vi "Advanced Functionality with Attributes.vi"() -> ()   [LabVIEW 2023]
doc: "The Advanced Functionality with Attributes example allows the user to view a camera's current attributes and settings, update attribute settings, acquire images continuously, and display the images in an image control. Note that the writeability of some attributes changes while acquiring and this is denoted by disabling the attribute."
uses:
  <vilib>/userdefined/High Color/IMAQdx.ctl
  <vilib>/vision/driver/IMAQdx.llb/IMAQdx Buffer Number Mode.ctl
  <vilib>/vision/driver/NI_Vision_Acquisition_Software.lvlib
panel:
  out "Frame Rate":dbl format="%#.2g"
  in  "Tab Control":T1(tab)
  in  "U32 Value Control":u32(slide) min=1 max=32768 step=1 scale=1.0..32768.0
  in  "DBL Value Control":dbl(slide) min=-100.0 max=100.0 step=1.0 scale=-100.0..100.0
  in  "String Value Control":string
  in  "Enum Value Control":u32(ring) items=["Mono8", "Mono10", "Mono12", "Mono14", "Mono16", "YUV422Packed"]
  in  "Boolean Value Control":bool
  in  "Command Value Control":bool
  in  "Grab":bool
  out "Tooltip":string
  out "Units":string
  in  "Attribute Tree":string(tree)
  out "Image":T2(plugin-control)
  out "Buffer Number":u32
  in  "Camera Name":refnum<k21> caption="IMAQdx Session"
  in  "Stop":bool
  # "Overview: Demonstrates how to view a camera's current attributes and settings, update attribute settings, acquire images continuously, and display the images in an image control.\nRequirements: Vision Acquisition Software\nInstructions: \n1. Select the Camera Name\n2. Run the VI\n3. Select various attributes in the tree to view the settings for the attribute.\n4. Press the Start Grab button and notice some attributes are no longer writeable; they are disabled. This is a property of attributes that can change as the acquisition state changes or other attribute values change."
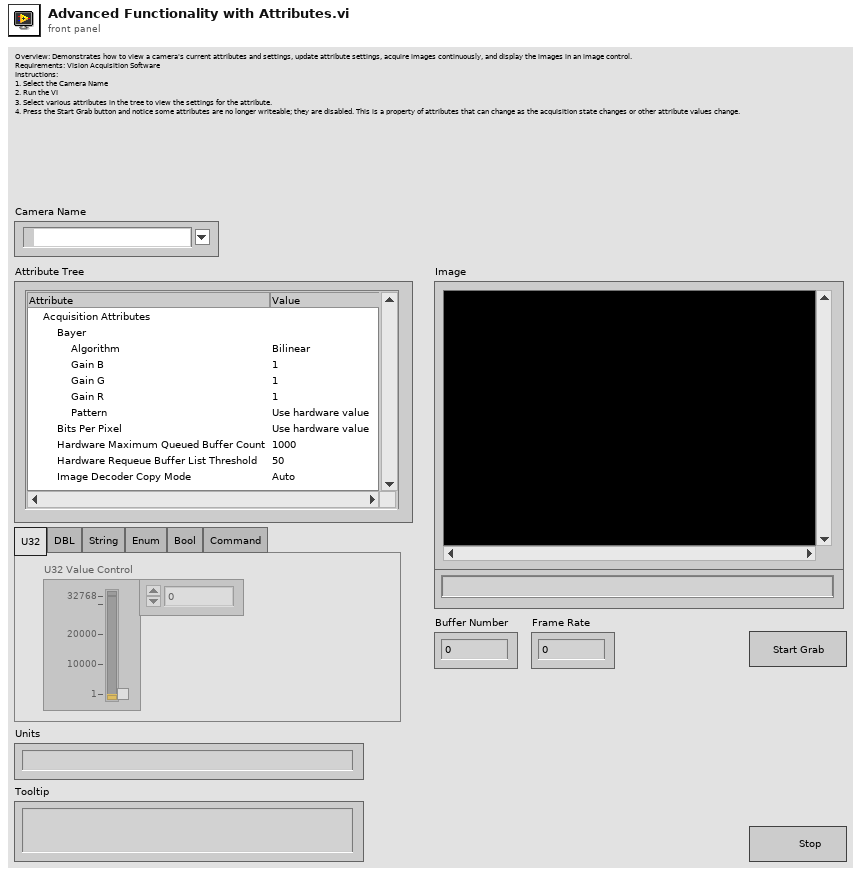
[diagram p1: front panel]
types:
  T1 = enum32{"U32", "DBL", "String", "Enum", "Bool", "Command"}
  T2 = typedef "IMAQ Image.ctl" = refnum<image>
  T3 = typedef "IMAQdx.ctl" = refnum<k21>
  T4 = cluster{"Tab Control":refnum<vi>, "U32 Value Control":refnum<vi>, "DBL Value Control":refnum<vi>, "String Value Control":refnum<vi>, "Enum Value Control":refnum<vi>, "Boolean Value Control":refnum<vi>, "Command Value Control":refnum<vi>}
  T5 = typedef "NI_Vision_Acquisition_Software.lvlib/IMAQdx Buffer Number Mode.ctl" = enum32{"Next", "Last", "Buffer Number", "Every", "Last New"}
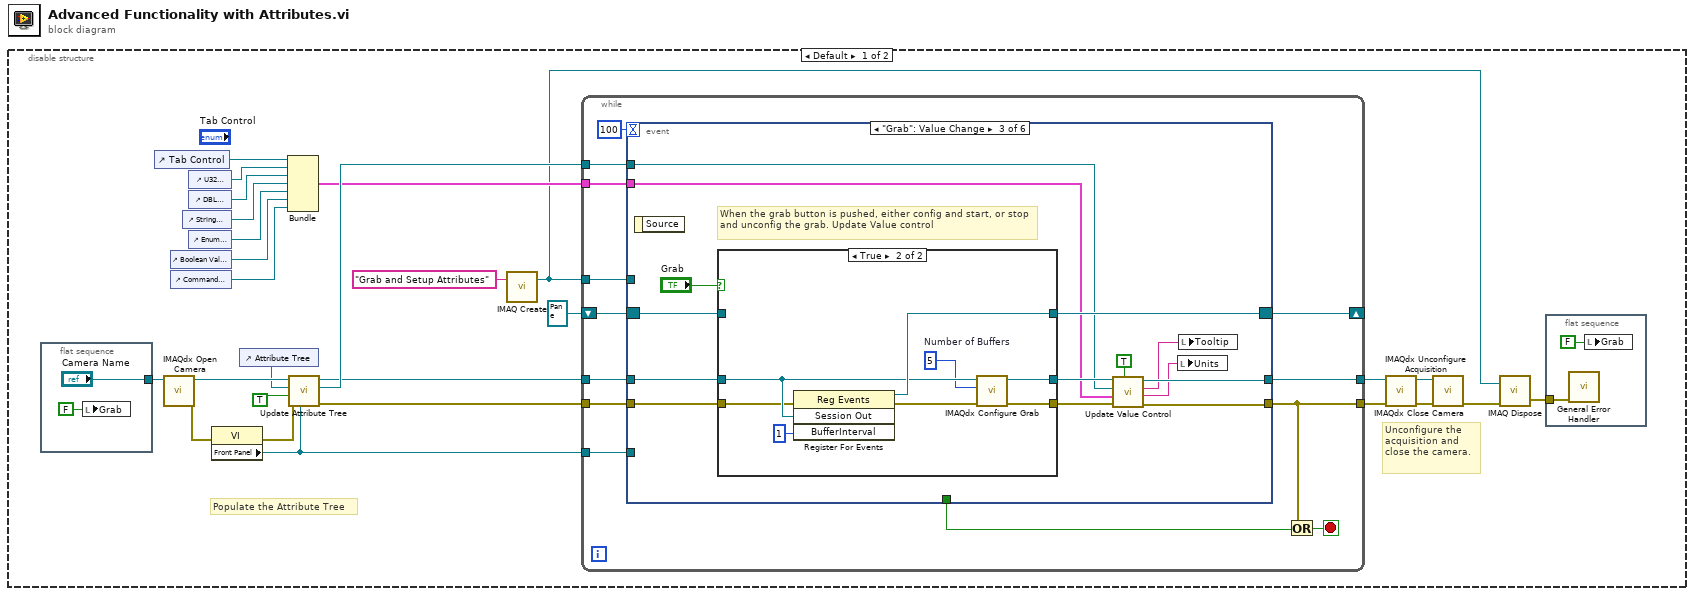
[diagram p0: block diagram]
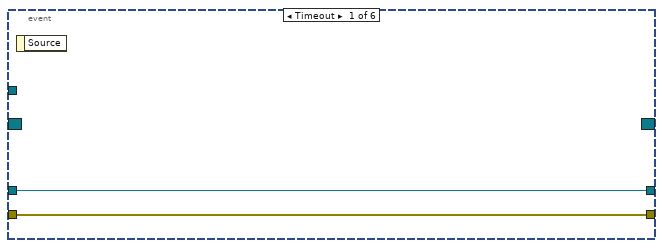
[diagram p2: hidden frame]
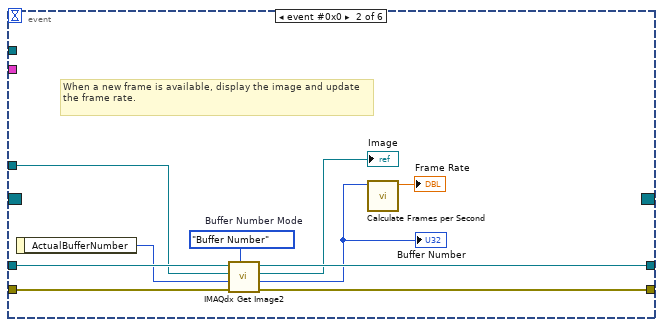
[diagram p3: hidden frame]
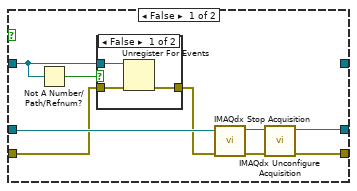
[diagram p4: hidden frame]
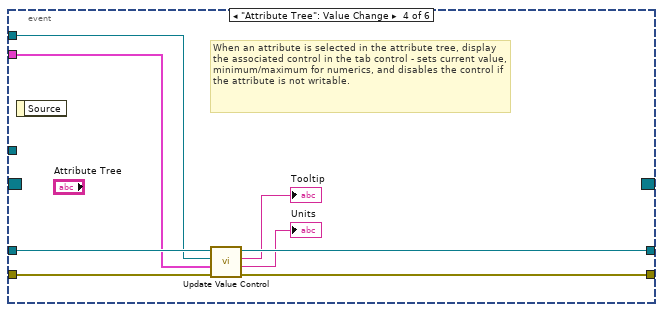
[diagram p6: hidden frame]
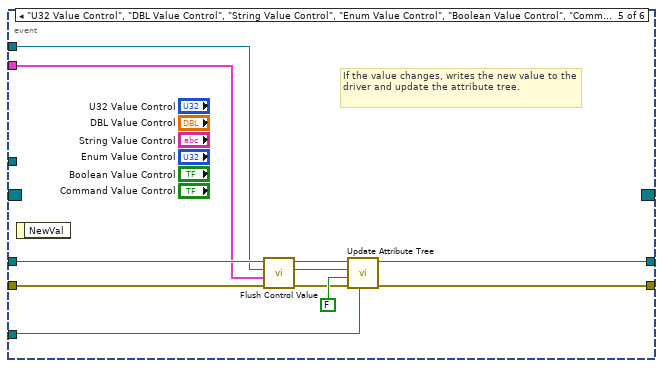
[diagram p7: hidden frame]
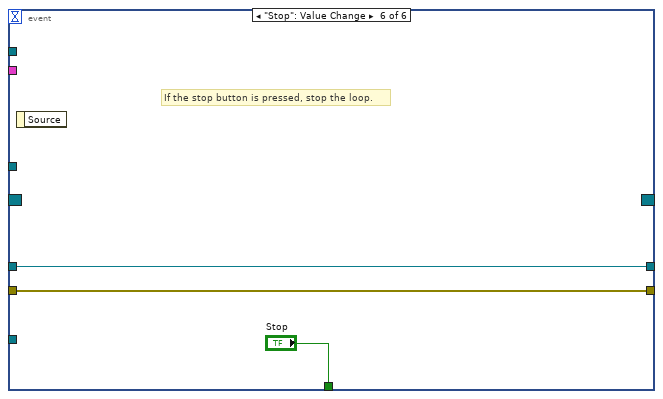
[diagram p8: hidden frame]
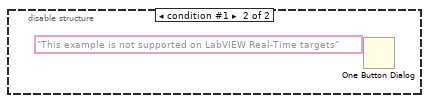
[diagram p9: hidden frame]
diagram:
  n1 = disable-structure shown="Default" {
    frame condition #0 (active) {
      # "Unconfigure the acquisition and close the camera."
      # "Populate the Attribute Tree"
      n2 = flat-sequence {
        tunnel: ["Camera Name"] -> w27
        frame #0 {
          n3 = local write "Grab"(FALSE ("Grab")) -> ()
        }
      }
      n4 = control-ref of="Tab Control"() -> (w7:refnum<vi>)
      n5 = call <vilib>:"IMAQdx Open Camera.vi"("Session In"=w27) -> ("error out"=w14:errorcluster, "Session Out"=w18:T3)  [unwired: 2 in, 7 out]
      n6 = control-ref of="Boolean Value Control"() -> (w20:refnum<vi>)
      n7 = control-ref of="Command Value Control"() -> (w19:refnum<vi>)
      n8 = control-ref of="String Value Control"() -> (w24:refnum<vi>)
      n9 = control-ref of="U32 Value Control"() -> (w23:refnum<vi>)
      n10 = control-ref of="DBL Value Control"() -> (w22:refnum<vi>)
      n11 = control-ref of="Enum Value Control"() -> (w21:refnum<vi>)
      n12 = property class="VI"(error in=w14) -> (error out=w6:errorcluster, "Front Panel"=w5:refnum<vi>)  [unwired: 1 in, 1 out]
      n13 = control-ref of="Attribute Tree"() -> (w17:refnum<vi>)
      n14 = Bundle("Tab Control"=w7, "U32 Value Control"=w23, "DBL Value Control"=w22, "String Value Control"=w24, "Enum Value Control"=w21, "Boolean Value Control"=w20, "Command Value Control"=w19) -> (w11:T4)  [unwired: 1 out]
      n15 = call "Update Attribute Tree.vi"("Panel Refnum In"=w5, "error in"=w6, "Flush Tree?"=TRUE, "Tree Control In"=w17, "Camera Name In"=w18) -> ("error out"=w3:errorcluster, "Tree Control Out"=w15:refnum<vi>, "Session Out"=w4:T3)  [unwired: 4 in]
      n16 = call "IMAQ Create"("Image Name"="Grab and Setup Attributes") -> ("New Image"=w9:T2)  [unwired: 3 in, 2 out]
      n17 = while {
        tunnel: [w40] -> w13
        tunnel: w3 -> [w42]
        tunnel: w4 -> [w43]
        tunnel: [w34] -> w12
        tunnel: w9 -> [w41]
        tunnel: w15 -> [w38]
        tunnel: w5 -> [w37]
        shift-right: [w35] -> _
        shift-left: refnum<event-registration> refnum ("Event Registration Refnum") -> [w39]
        tunnel: w11 -> [w33]
        stop <- w44 stop-if-true
        n18 = event shown="[2] \"Grab\": Value Change" {
          selector: w39 -> [_ _ w57 _ _ _]
          dyn-events: [_ _ w68 _ _ _] -> w35
          timeout: 100 -> [_ _ _ _ _ _]
          tunnel: w43 -> [w45 w56 w70 w99 w109 w111]
          tunnel: w42 -> [w46 w55 w67 w97 w110 w112]
          tunnel: w41 -> [_ w54 _ _ _ _]
          tunnel: [w45 w53 w60 w98 w105 w111] -> w40
          tunnel: [w46 w52 w64 w96 w101 w112] -> w34
          tunnel: w38 -> [_ _ w63 w94 w103 _]
          tunnel: w37 -> [_ _ _ _ w100 _]
          tunnel: [_ _ _ _ _ "Stop"] -> w36
          tunnel: w33 -> [_ _ w61 w95 w104 _]
          event Timeout {
            n19 = event-data() -> ()  [unwired: 2 out]
          }
          event event #0x0 {
            w50 = IMAQdx_Buffer_Number_Mode."Buffer Number"  # Buffer Number Mode
            # "When a new frame is available, display the image and update the frame rate."
            n20 = event-data() -> ("ActualBufferNumber"=w49:u32)  [unwired: 1 out]
            n21 = call <vilib>:"IMAQdx Get Image2.vi"("Buffer Number Mode (Next)"=w50, "error in"=w55, "Buffer Number In"=w49, "Image In"=w54, "Session In"=w56) -> ("error out"=w52:errorcluster, "Buffer Number Out"=w48:u32, "Image Out"=→"Image":T2, "Session Out"=w53:T3)  [unwired: 3 in]
            "Buffer Number" <- w48
            n22 = call <vilib>:"Calculate Frames per Second.vi"("Buffer Number"=w48) -> ("Acquired Frames/s"=→"Frame Rate":dbl)  [unwired: 8 in, 2 out]
          }
          event "Grab": Value Change {
            # "When the grab button is pushed, either config and start, or stop and unconfig the grab. Update Value control"
            n23 = event-data() -> ()  [unwired: 2 out]
            n24 = case shown="True" "Grab" {
              tunnel: w70 -> [w79 w89]
              tunnel: [w76 w85] -> w66
              tunnel: [w75 w86] -> w65
              tunnel: [_ w91] -> w68
              tunnel: w57 -> [w72 _]
              tunnel: w67 -> [w73 w88]
              frame False {
                n25 = Not A Number/Path/Refnum?(number/path/refnum=w72) -> (NaN/Path/Refnum?=w71:bool)
                n26 = case shown="False" w71 {
                  tunnel: [w82 w83] -> w74
                  tunnel: w73 -> [w81 w83]
                  tunnel: w72 -> [w80 _]
                  frame False {
                    n27 = Unregister For Events(event registration refnum=w80, error in=w81) -> (error out=w82:errorcluster)
                  }
                  frame True {
                  }
                }
                n28 = call <vilib>:"IMAQdx Stop Acquisition.vi"("error in"=w74, "Session In"=w79) -> ("error out"=w77:errorcluster, "Session Out"=w78:T3)  [unwired: 8 out]
                n29 = call <vilib>:"IMAQdx Unconfigure Acquisition.vi"("error in"=w77, "Session In"=w78) -> ("error out"=w75:errorcluster, "Session Out"=w76:T3)  [unwired: 8 out]
              }
              frame True {
                w84 = u32 5  # Number of Buffers
                n30 = register-events(error in=w88, w89, u32 1 ("BufferInterval")) -> (reference out=w91:refnum<event-registration>, error out=w87:errorcluster)  [unwired: 1 in]
                n31 = call <vilib>:"IMAQdx Configure Grab.vi"("error in"=w87, "Number of Buffers"=w84, "Session In"=w89) -> ("error out"=w86:errorcluster, "Session Out"=w85:T3)  [unwired: 7 in]
              }
            }
            n32 = call "Update Value Control.vi"("Force update?"=TRUE, "error in (no error)"=w65, "Tab Control Ref In"=w61, "Tree Control In"=w63, "Session In"=w66) -> ("error out"=w64:errorcluster, "Units"=w58:string, "Tooltip"=w59:string, "Session Out"=w60:T3)  [unwired: 3 in]
            n33 = local write "Units"(w58) -> ()
            n34 = local write "Tooltip"(w59) -> ()
          }
          event "Attribute Tree": Value Change {
            # "When an attribute is selected in the attribute tree, display the associated control in the tab control - sets current value, minimum/maximum for numerics, and disables the control if the attribute is not writable."
            n35 = event-data() -> ()  [unwired: 2 out]
            n36 = call "Update Value Control.vi"("error in (no error)"=w97, "Tab Control Ref In"=w95, "Tree Control In"=w94, "Session In"=w99) -> ("error out"=w96:errorcluster, "Units"=→"Units":string, "Tooltip"=→"Tooltip":string, "Session Out"=w98:T3)  [unwired: 4 in]
          }
          event "U32 Value Control", "DBL Value Control", "String Value Control", "Enum Value Control", "Boolean Value Control", "Command Value Control": Value Change {
            # "If the value changes, writes the new value to the driver and update the attribute tree."
            n37 = event-data() -> ()  [unwired: 2 out]
            n38 = call "Flush Control Value.vi"("error in (no error)"=w110, "Tab Control Ref In"=w104, "Tree Control In"=w103, "Session In"=w109) -> ("error out"=w102:errorcluster, "Tree Control Out"=w107:refnum<vi>, "Session Out"=w108:T3)  [unwired: 5 in]
            n39 = call "Update Attribute Tree.vi"("Panel Refnum In"=w100, "error in"=w102, "Flush Tree?"=FALSE, "Tree Control In"=w107, "Camera Name In"=w108) -> ("error out"=w101:errorcluster, "Session Out"=w105:T3)  [unwired: 4 in, 1 out]
          }
          event "Stop": Value Change {
            # "If the stop button is pressed, stop the loop."
            n40 = event-data() -> ()  [unwired: 2 out]
          }
        }
        n41 = Or(x=w34, y=w36) -> (x .or. y?=w44:bool)
      }
      n42 = call <vilib>:"IMAQdx Unconfigure Acquisition.vi"("error in"=w12, "Session In"=w13) -> ("error out"=w26:errorcluster, "Session Out"=w25:T3)  [unwired: 8 out]
      n43 = call <vilib>:"IMAQdx Close Camera.vi"("error in"=w26, "Session In"=w25) -> ("error out"=w10:errorcluster)  [unwired: 9 out]
      n44 = call "IMAQ Dispose"("Image"=w9, "error in (no error)"=w10) -> ("error out"=w1:errorcluster)  [unwired: 4 in]
      n45 = flat-sequence {
        tunnel: w1 -> [w29]
        frame #0 {
          n46 = call <vilib>:"General Error Handler.vi"("error in (no error)"=w29) -> ()  [unwired: 2 in, 13 out]
          n47 = local write "Grab"(FALSE ("Grab")) -> ()
        }
      }
    }
    frame condition #1 {
      n48 = One Button Dialog(message="This example is not supported on LabVIEW Real-Time targets" ("source")) -> ()  [unwired: 1 in, 1 out]
    }
  }
